vi "Change Button Color.vi"(8 "error in (no error)":errorcluster, 10 "Colors [4]":cluster{u32, u32}[](array[cluster]), 11 "Button in":refnum<class "Button.lvclass">) -> (0 "error out":errorcluster, 3 "Button out":refnum<class "Button.lvclass">)   [LabVIEW 2018, in "Button.lvclass"]
uses:
  callbuttonv1.1/Button Class/Button.lvclass
panel:
  in  "stop":bool
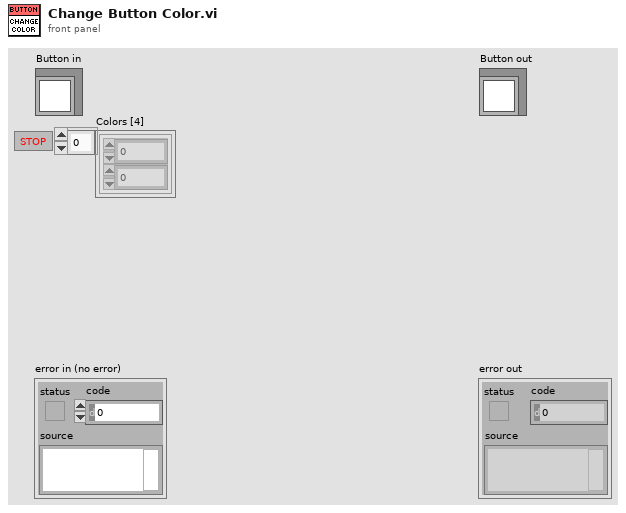
[diagram p1: front panel]
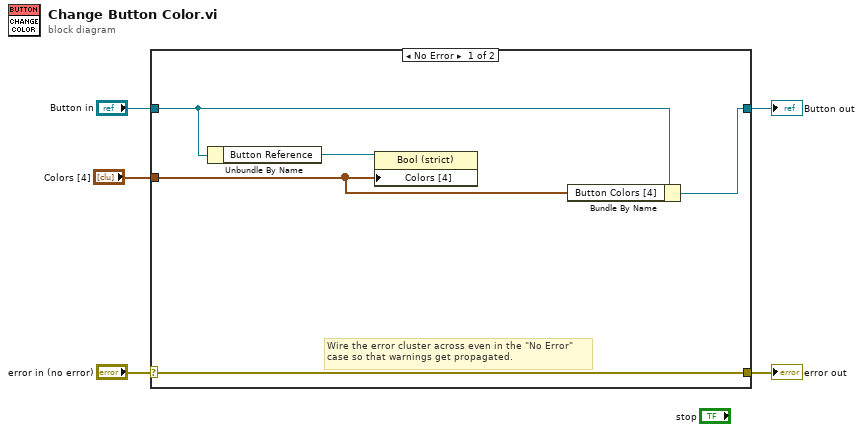
[diagram p0: block diagram]
diagram:
  n1 = case shown="No Error" "error in (no error)" {
    selector: "error in (no error)" -> [w10 w12]
    tunnel: [w10 w12] -> w4
    tunnel: [w7 w11] -> w2
    tunnel: "Button in" -> [w8 w11]
    tunnel: "Colors [4]" -> [w6 _]
    frame No Error {
      # "Wire the error cluster across even in the \"No Error\"\ncase so that warnings get propagated."
      n2 = Unbundle By Name(w8) -> ("Button Reference"=w9:refnum<vi>)
      n3 = property class="Bool (strict)"(reference=w9, "Colors [4]"=w6) -> ()  [unwired: 1 in, 2 out]
      n4 = Bundle By Name(cluster=w8, "Button Colors [4]"=w6) -> (w7:refnum<class "Button.lvclass">)
    }
    frame Error {
    }
  }
  "error out" <- w4
  "Button out" <- w2
